vi "Create Data File.vi"(8 "错误输入":cluster{"状态":bool, "代码":i32, "源":string}) -> (0 "错误输出":cluster{"状态":bool, "代码":i32, "源":string}, 3 "文件引用句柄":refnum<file>)   [LabVIEW 2012]
doc: "本VI通过执行一系列任务，为记录数据创建一个文件：\n\n1) 检查应用程序目录下是否存在名称为Logged Data的文件夹\n2) 如不存在，则创建该文件夹\n3) 按“采集数据 <日期> <时间>.txt”格式，生成一个文件名称\n4) 替换或创建文件"
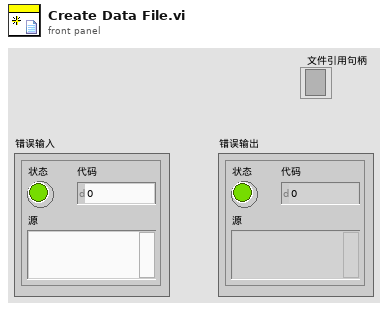
[diagram p1: front panel]
types:
  T1 = enum16{"open", "replace", "create", "open or create", "replace or create", "replace or create with confirmation"}
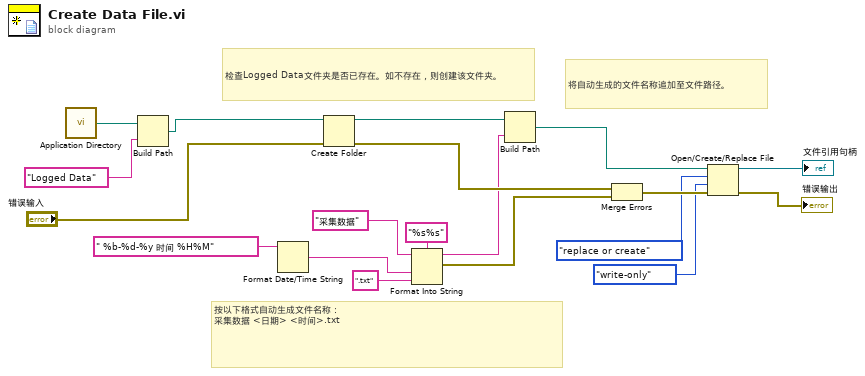
[diagram p0: block diagram]
diagram:
  # "将自动生成的文件名称追加至文件路径。"
  # "检查Logged Data文件夹是否已存在。如不存在，则创建该文件夹。"
  # "按以下格式自动生成文件名称：\n采集数据 <日期> <时间>.txt"
  n1 = call <vilib>:"Application Directory.vi"() -> ("Application Directory"=w10:path)
  n2 = Build Path ("创建路径")(base path=w10, name or relative path="Logged Data" ("对话框窗口（创建文件夹）")) -> (appended path=w2:path)
  n3 = Format Date/Time String ("格式化日期/时间字符串")(time format string (%c)=" %b-%d-%y 时间 %H%M" ("时间格式字符串(%c)")) -> (date/time string=w6:string)  [unwired: 2 in]
  n4 = Create Folder ("创建文件夹")(path (use dialog)=w2, error in="错误输入") -> (created path=w13:path, error out=w12:errorcluster)  [unwired: 1 in, 1 out]
  n5 = Format Into String ("格式化写入字符串")(format string="%s%s" ("格式字符串"), initial string="采集数据" ("字符串"), w6, ".txt" ("字符串")) -> (resulting string=w3:string, error out=w4:errorcluster)  [unwired: 1 in]
  n6 = Build Path ("创建路径")(base path=w13, name or relative path=w3) -> (appended path=w19:path)
  n7 = Merge Errors ("合并错误")(w12, w4) -> (w18:errorcluster)
  n8 = Open/Create/Replace File ("打开/创建/替换文件")(file path (use dialog)=w19, error in=w18, operation (0:open)=T1."replace or create" ("操作(0:open)"), access (0:read/write)=enum16{"read/write", "read-only", "write-only"}."write-only" ("权限(0:read/write)")) -> (refnum out=→"文件引用句柄":refnum<file>, error out=→"错误输出":errorcluster)  [unwired: 2 in, 1 out]
